vi "UDS(State).vi"() -> ()   [LabVIEW 2020]
uses:
  <vilib>/Automotive Diagnostic Command Set/Diagnostic Transport.llb/Transport Protocol Selector.ctl
  <vilib>/Automotive Diagnostic Command Set/Diagnostic Transport.llb/Property ID.ctl
  <vilib>/Automotive Diagnostic Command Set/Diagnostic Transport.llb/Diag Reference.ctl
  <vilib>/Automotive Diagnostic Command Set/Diagnostic Transport.llb/DoIP Protocol Version.ctl
  <vilib>/Automotive Diagnostic Command Set/Diagnostic Transport.llb/Diag Globals.ctl
  <vilib>/addons/Automotive Diagnostic Command Set/NI_Automotive Diagnostic Command Set.lvlib
panel:
  out "Clear DTC":bool
  out "Finish":bool
  out "Auto?":bool
  in  "Auto":bool
  in  "Reset":bool
  out "CAN_log":string[][](table)
  out "Response":u8[](array[numeric]) format="%.0x"
  in  "Close":bool
  in  "Stop":bool
  in  "Start":bool
  in  "Option":i32(ring) items=["读软件版本", "读DTC", "清DTC"]
  in  "Action":bool
  out "open_ok?":bool
  # "读软件版本→读写DTC→ 清DTC log→读软件版本→读写DTC→ 清DTC log\n运行程序，点击“Start”，Open Diagnostic\nOption：选择需要的操做；Write：手动发送指令；\nReset：清除表格内容；\nAuto：自动按照上面所要求顺序进行读写操作；\nClose：Close Diagnostic；\nStop：停止程序。"
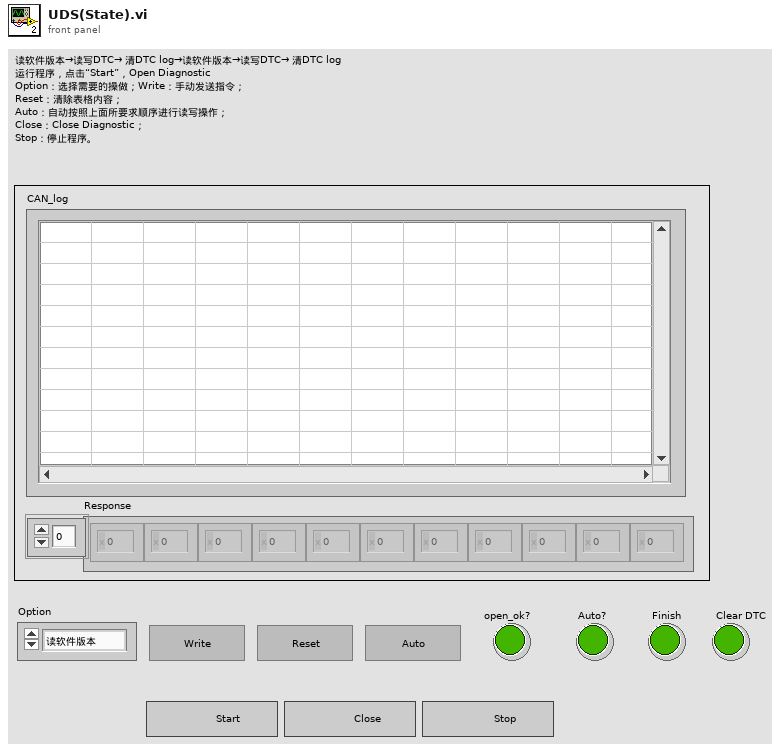
[diagram p1: front panel]
types:
  T1 = typedef "NI_Automotive Diagnostic Command Set.lvlib/Property ID.ctl" = enum16{"Timeout Diag Command", "Timeout FC (Bs)", "Timeout CF (Cr)", "Receive Block Size (BS)", "Wait Time CF (STmin)", "Max Wait Frames (N_WFTmax)", "Wait Frames to Send (N_WAIT)", "Time between Waits (T_W)", "Fill CAN Frames", "Fill Byte", "Invalid Response as Error", "Max RspPending Count", "VWTP Command Timeout", "STmin", "P2min", "Termination", "Timeout RspPending", "LIN Sleep", "Actual CAN IO Mode", "Response Plausibility Check", "Session-based Properties"}
  T2 = typedef "NI_Automotive Diagnostic Command Set.lvlib/Transport Protocol Selector.ctl" = enum16{"ISO TP - Normal Mode", "ISO TP - Mixed Mode", "VW TP 2.0", "Diagnostics on IP", "ISO TP LIN"}
  T3 = typedef "NI_Automotive Diagnostic Command Set.lvlib/Diag Reference.ctl" = cluster{"Diag CAN Handle":u32, "Transport Protocol":T2, "Receive Address Extension":u8, "Transmit Address Extension":u8, "Receive CAN Id":u32, "Transmit CAN Id":u32, "Log Frames ?":bool, "My TP Address":u8, "Other TP Address":u8, "T1":u16, "T2":u16, "T3":u16, "T4":u16, "Tx SN":u8, "Block Size":u8, "Rx SN":u8, "VW TP Initialized?":bool, "Tx block no":u8, "baud rate":u64, "Interface":string, "Channel Diag CAN Handle":u32, "UDP Connection ID":refnum<k16>, "TCP Connection ID":refnum<k5>, "Target IP Addr":u32, "Source Address":u16, "Target Address":u16, "Send Header NACK?":bool, "DLL Handle":u32, "NAD":u8, "Time Stamp read first":dbl, "Time Stamp read last":dbl, "Time Stamp write first":dbl, "Time Stamp write last":dbl, "Time Stamp write":dbl, "Time Stamp read":dbl, " I/O Mode":u32, "FD Baudrate":u64, "TX_DL":u16, "RX_DL":u16, "DoIP Protocol Version":T4, " Selected I/O Mode":u32, "TesterPresent Counter":u32, "TesterPresent Limit":u32, "TesterPresent Tick[ms]":i32, "TesterPresent RequireResponse?":bool, "TesterPresent Stored Ref?":bool, "TesterPresent Message":u8[], "TesterPresent Task Handle":i32, "TesterPresent Semaphore":T5, "Response Plausibility Check":u32, "Default Version?":bool, "Diagostic Globals":T6, "Session-based Properties?":bool}
  T4 = typedef "NI_Automotive Diagnostic Command Set.lvlib/DoIP Protocol Version.ctl" = u8
  T5 = typedef "Semaphore RefNum" = refnum<k1>
  T6 = typedef "NI_Automotive Diagnostic Command Set.lvlib/Diag Globals.ctl" = cluster{"Timeout FC (Bs)":u32, "Timeout CF (Cr)":u32, "Timeout Diag Command":u32, "Receive Block Size (BS)":u8, "Wait Time CF (STmin)":u8, "Max Waits (N_WFTmax)":u8, "Waits to Send (N_WAIT)":i32, "Time between Waits (TW)":u32, "Fill CAN Frames?":bool, "Fill Byte":u32, "Invalid Response as Error?":bool, "Max RspPending Count":u32, "VWTP Command Timeout":u32, "Transport Protocol":T2, "Diag CAN Handle":u32, "DLL Handle":u32, "Timeout RspPending":u32}
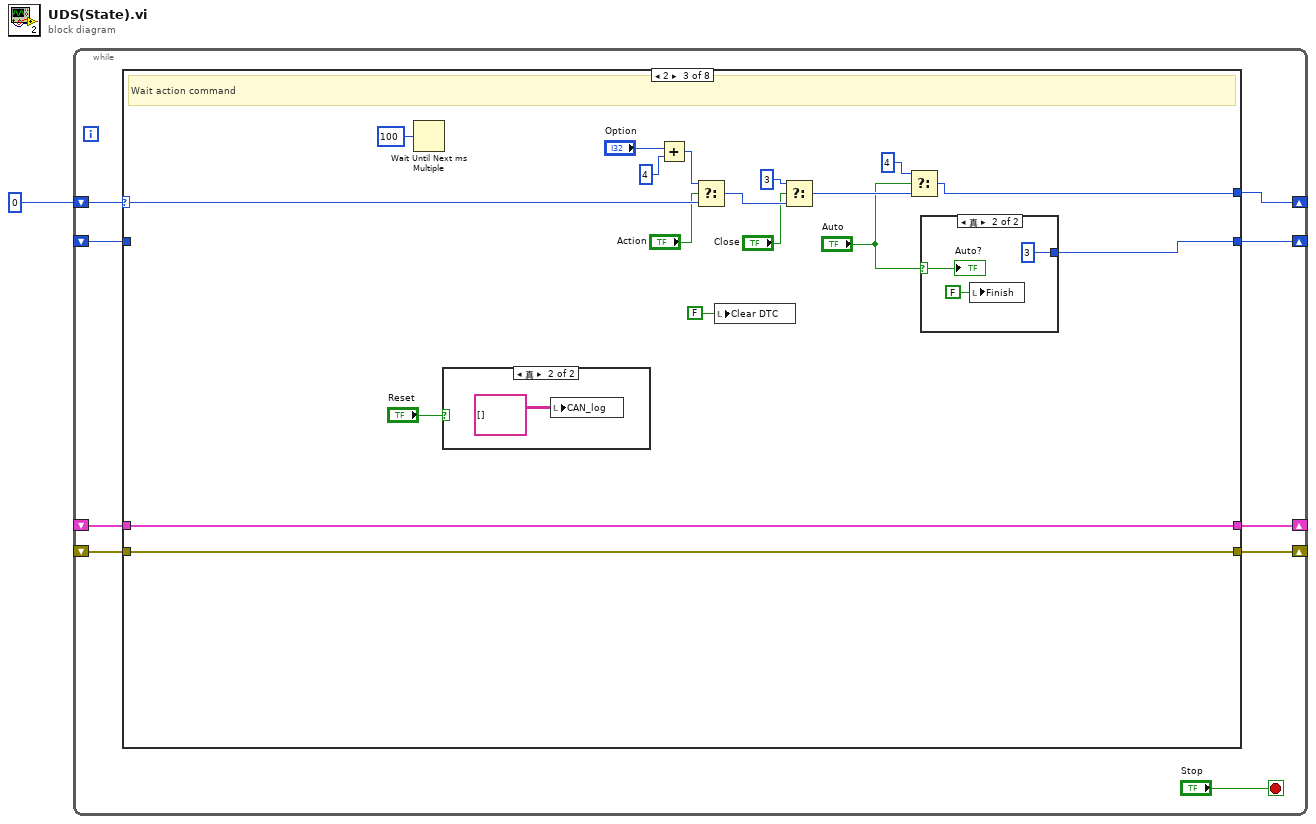
[diagram p0: block diagram]
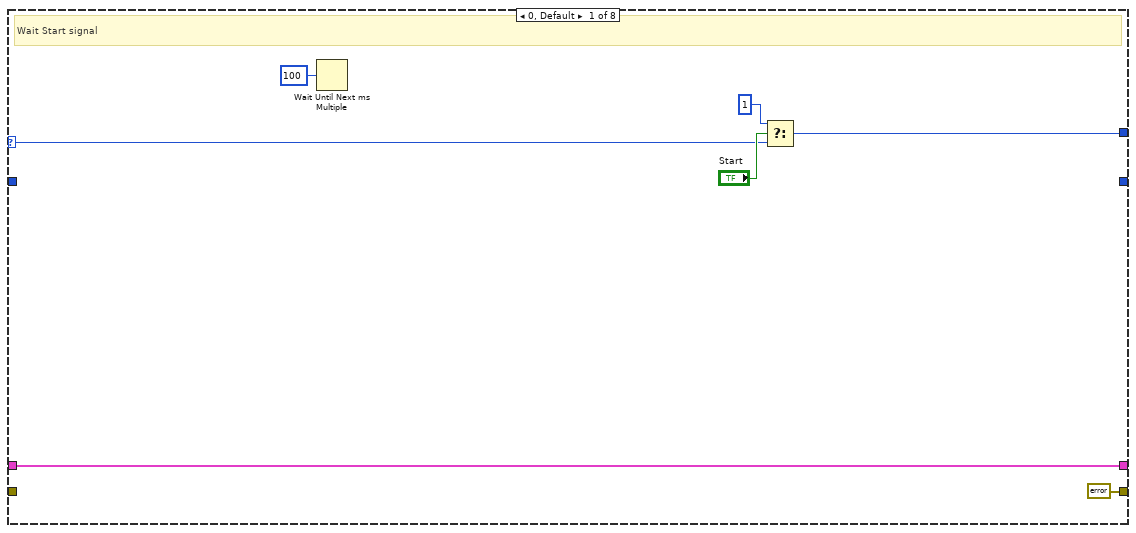
[diagram p2: hidden frame]
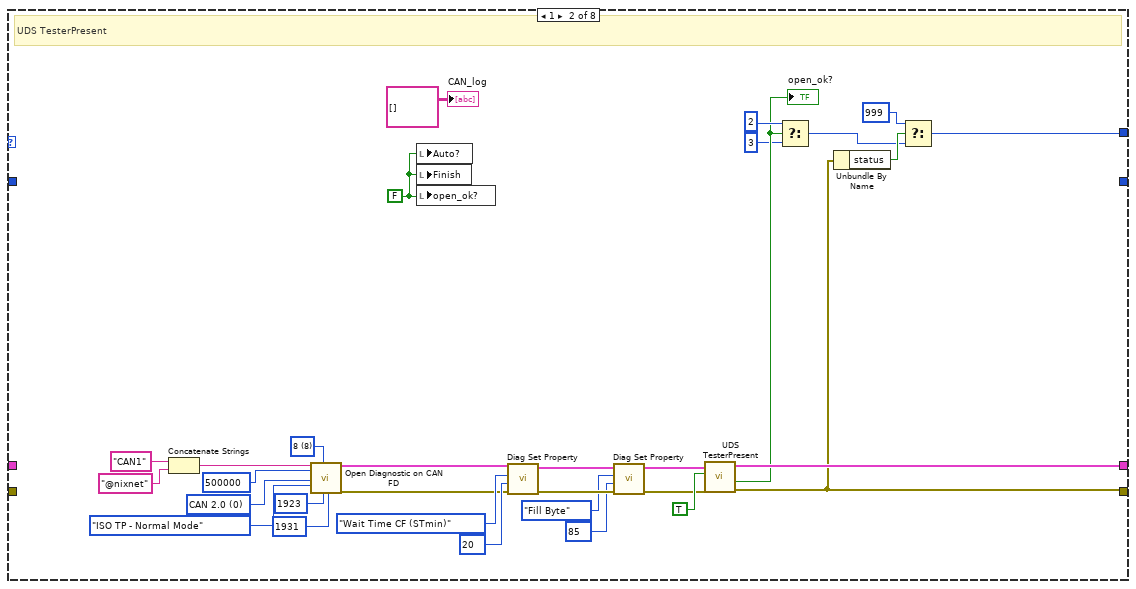
[diagram p3: hidden frame]
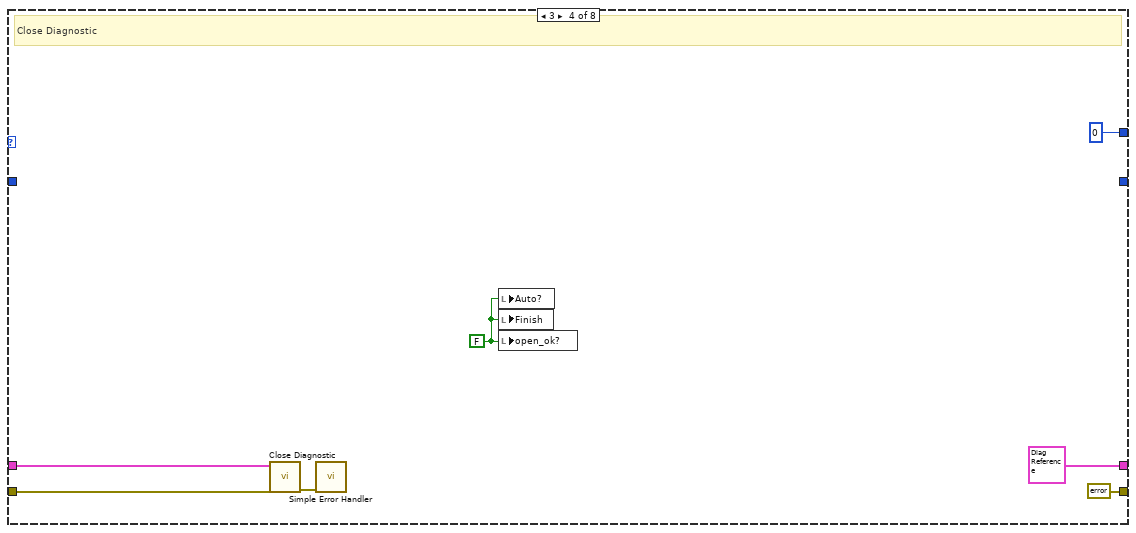
[diagram p6: hidden frame]
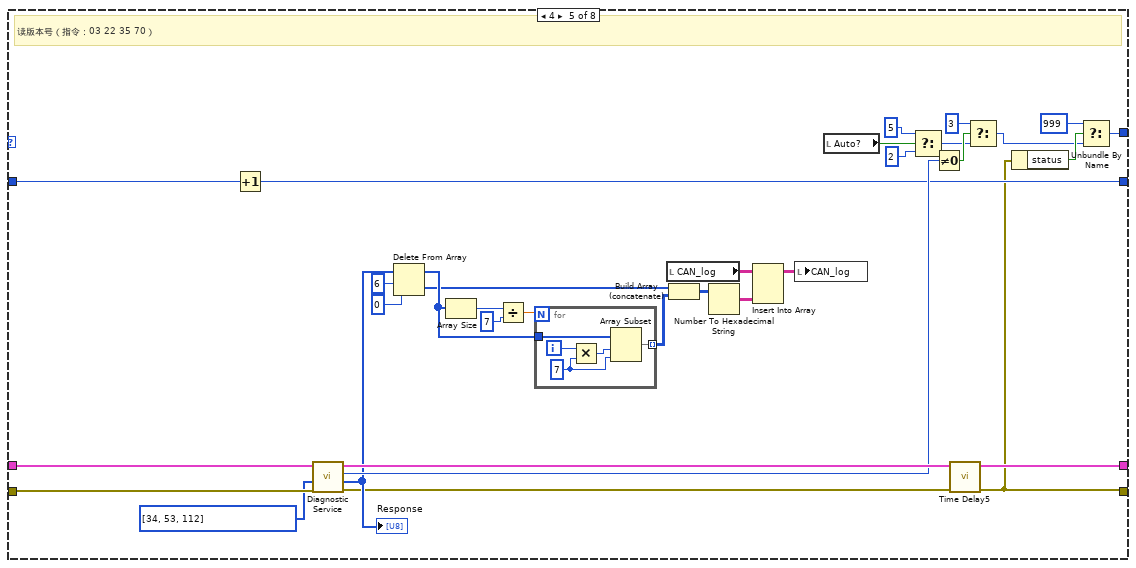
[diagram p7: hidden frame]
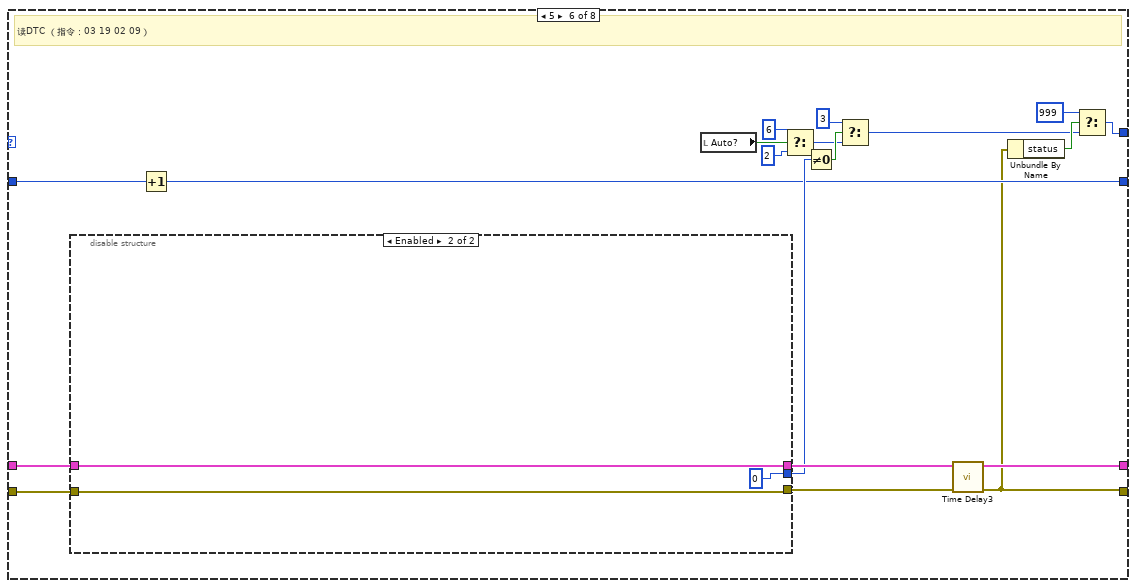
[diagram p8: hidden frame]
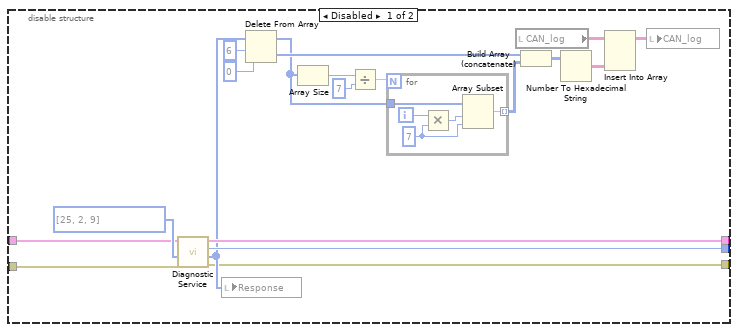
[diagram p9: hidden frame]
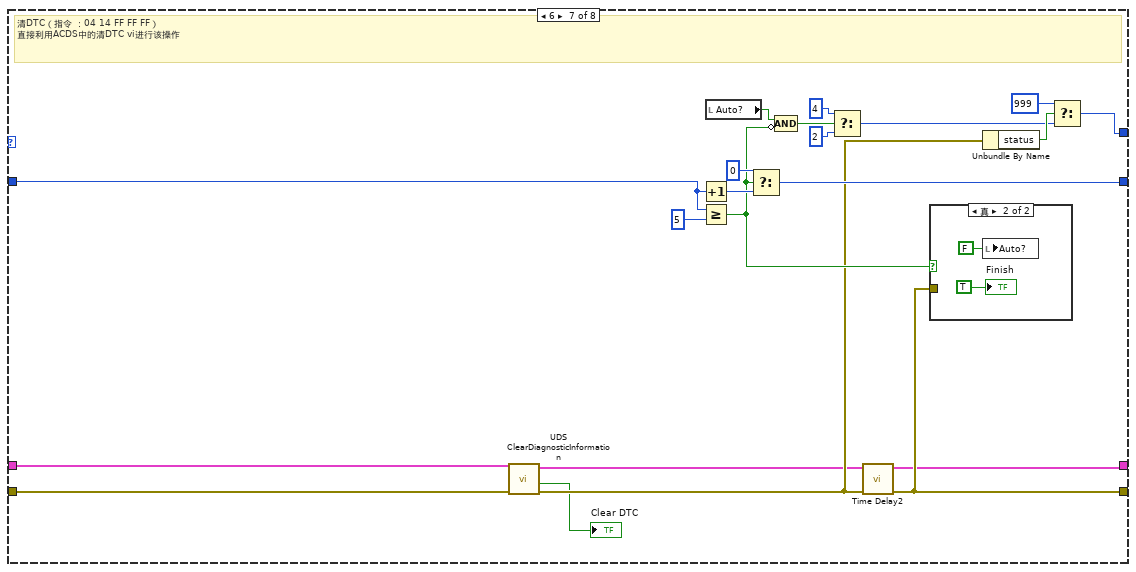
[diagram p10: hidden frame]
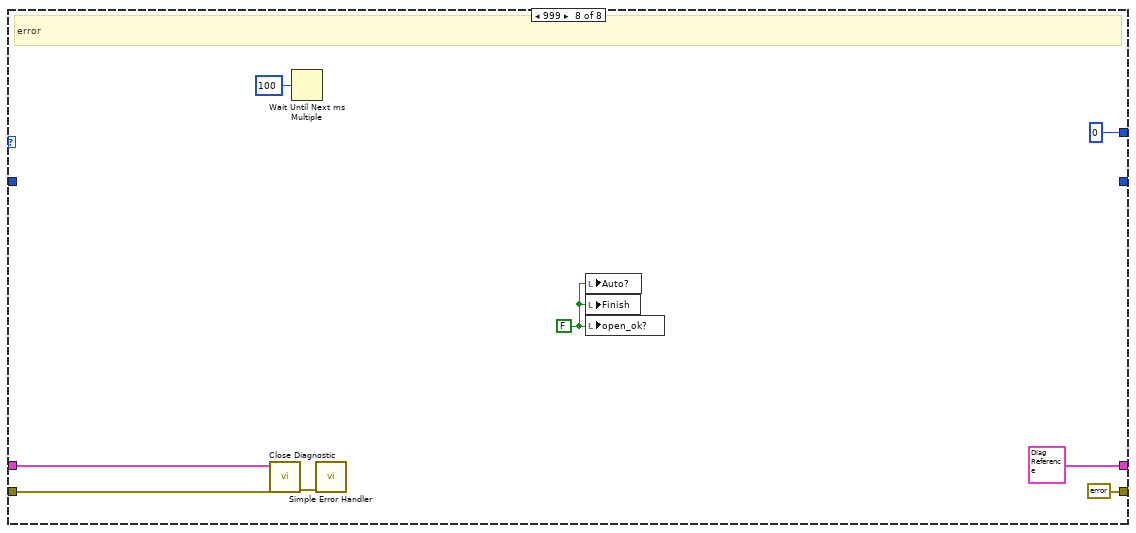
[diagram p12: hidden frame]
diagram:
  n1 = while {
    shift-right: [w5] -> _
    shift-left: 0 -> [w10]
    shift-right: [w7] -> _
    shift-left: _ -> [w9]
    shift-right: [w6] -> _
    shift-left: _ -> [w8]
    shift-right: [w3] -> _
    shift-left: _ -> [w2]
    stop <- "Stop" stop-if-true
    n2 = case shown="2" w10 {
      selector: w10 -> [w13 _ w66 _ _ _ _ _]
      tunnel: w9 -> [w17 _ w65 w75 w109 w131 w164 w187]
      tunnel: w8 -> [_ _ w64 w76 w81 w130 w163 w188]
      tunnel: [w17 w48 w65 T3 {"Diag CAN Handle"=0, "Transport Protocol"=enum."ISO TP - Normal Mode", "Receive Address Extension"=0, "Transmit Address Extension"=0, "Receive CAN Id"=0, "Transmit CAN Id"=0, "Log Frames ?"=FALSE, "My TP Address"=0, "Other TP Address"=0, "T1"=0, "T2"=0, "T3"=0, "T4"=0, "Tx SN"=0, "Block Size"=0, "Rx SN"=0, "VW TP Initialized?"=FALSE, "Tx block no"=0, "baud rate"=0, "Interface"="", "Channel Diag CAN Handle"=0, "UDP Connection ID"=refnum, "TCP Connection ID"=refnum, "Target IP Addr"=0, "Source Address"=0, "Target Address"=0, "Send Header NACK?"=FALSE, "DLL Handle"=0, "NAD"=0, "Time Stamp read first"=0.0, "Time Stamp read last"=0.0, "Time Stamp write first"=0.0, "Time Stamp write last"=0.0, "Time Stamp write"=0.0, "Time Stamp read"=0.0, " I/O Mode"=0, "FD Baudrate"=0, "TX_DL"=8, "RX_DL"=8, "DoIP Protocol Version"=1, " Selected I/O Mode"=0, "TesterPresent Counter"=0, "TesterPresent Limit"=0, "TesterPresent Tick[ms]"=10, "TesterPresent RequireResponse?"=FALSE, "TesterPresent Stored Ref?"=FALSE, "TesterPresent Message"=[], "TesterPresent Task Handle"=0, "TesterPresent Semaphore"=refnum, "Response Plausibility Check"=1, "Default Version?"=TRUE, "Diagostic Globals"={"Timeout FC (Bs)"=250, "Timeout CF (Cr)"=250, "Timeout Diag Command"=1000, "Receive Block Size (BS)"=0, "Wait Time CF (STmin)"=5, "Max Waits (N_WFTmax)"=10, "Waits to Send (N_WAIT)"=0, "Time between Waits (TW)"=25, "Fill CAN Frames?"=TRUE, "Fill Byte"=255, "Invalid Response as Error?"=FALSE, "Max RspPending Count"=5, "VWTP Command Timeout"=50, "Transport Protocol"=enum."Diagnostics on IP", "Diag CAN Handle"=0, "DLL Handle"=0, "Timeout RspPending"=1000}, "Session-based Properties?"=FALSE} ("diag ref out") w108 w129 w161 T3 {"Diag CAN Handle"=0, "Transport Protocol"=enum."ISO TP - Normal Mode", "Receive Address Extension"=0, "Transmit Address Extension"=0, "Receive CAN Id"=0, "Transmit CAN Id"=0, "Log Frames ?"=FALSE, "My TP Address"=0, "Other TP Address"=0, "T1"=0, "T2"=0, "T3"=0, "T4"=0, "Tx SN"=0, "Block Size"=0, "Rx SN"=0, "VW TP Initialized?"=FALSE, "Tx block no"=0, "baud rate"=0, "Interface"="", "Channel Diag CAN Handle"=0, "UDP Connection ID"=refnum, "TCP Connection ID"=refnum, "Target IP Addr"=0, "Source Address"=0, "Target Address"=0, "Send Header NACK?"=FALSE, "DLL Handle"=0, "NAD"=0, "Time Stamp read first"=0.0, "Time Stamp read last"=0.0, "Time Stamp write first"=0.0, "Time Stamp write last"=0.0, "Time Stamp write"=0.0, "Time Stamp read"=0.0, " I/O Mode"=0, "FD Baudrate"=0, "TX_DL"=8, "RX_DL"=8, "DoIP Protocol Version"=1, " Selected I/O Mode"=0, "TesterPresent Counter"=0, "TesterPresent Limit"=0, "TesterPresent Tick[ms]"=10, "TesterPresent RequireResponse?"=FALSE, "TesterPresent Stored Ref?"=FALSE, "TesterPresent Message"=[], "TesterPresent Task Handle"=0, "TesterPresent Semaphore"=refnum, "Response Plausibility Check"=1, "Default Version?"=TRUE, "Diagostic Globals"={"Timeout FC (Bs)"=250, "Timeout CF (Cr)"=250, "Timeout Diag Command"=1000, "Receive Block Size (BS)"=0, "Wait Time CF (STmin)"=5, "Max Waits (N_WFTmax)"=10, "Waits to Send (N_WAIT)"=0, "Time between Waits (TW)"=25, "Fill CAN Frames?"=TRUE, "Fill Byte"=255, "Invalid Response as Error?"=FALSE, "Max RspPending Count"=5, "VWTP Command Timeout"=50, "Transport Protocol"=enum."Diagnostics on IP", "Diag CAN Handle"=0, "DLL Handle"=0, "Timeout RspPending"=1000}, "Session-based Properties?"=FALSE} ("diag ref out")] -> w7
      tunnel: [errorcluster {"status"=FALSE, "code"=0, "source"=""} ("error out") w35 w64 errorcluster {"status"=FALSE, "code"=0, "source"=""} ("error out") w79 w115 w165 errorcluster {"status"=FALSE, "code"=0, "source"=""} ("error out")] -> w6
      tunnel: [w12 w31 w51 0 ("t") w95 w117 w166 0 ("t")] -> w5
      tunnel: [_ _ w52 _ w101 w122 w177 _] -> w3
      tunnel: w2 -> [_ _ _ _ w100 w123 w176 _]
      frame 0, Default {
        # "Wait Start signal"
        n3 = Wait Until Next ms Multiple(millisecond multiple=u32 100) -> ()  [unwired: 1 out]
        n4 = Select(t=1, s="Start", f=w13) -> (s? t:f=w12:i32)
      }
      frame 1 {
        w29 = FALSE ("success?")
        w41 = u16 8 items=["8"=8, "12"=12, "16"=16, "20"=20, "24"=24, "32"=32, "48"=48, "64"=64] ("Max DLC")
        w43 = u32 0 items=["CAN 2.0", "CAN FD", "CAN FD+BRS", "ECU Determined"] ("IO Mode")
        # "UDS TesterPresent"
        n5 = Concatenate Strings("CAN1" ("Name"), "@nixnet") -> (w45:string)
        n6 = call <vilib>:"Open Diagnostic on CAN FD.vi"("CAN Interface"=w45, "Baud Rate"=u64 500000, "IO Mode"=w43, "Transport Protocol"=Transport_Protocol_Selector."ISO TP - Normal Mode", "Max DLC"=w41, "Transmit ID"=u32 1923, "Receive ID"=u32 1931) -> ("diag ref out"=w21:T3, "error out"=w19:errorcluster)  [unwired: 11 in]
        n7 = local write "Auto?"(w29) -> ()
        n8 = local write "Finish"(w29) -> ()
        n9 = local write "open_ok?"(w29) -> ()
        n10 = call <vilib>:"Diag Set Property.vi"("error in (no error)"=w19, "property value"=u32 20, "property ID"=Property_ID."Wait Time CF (STmin)", "diag ref in"=w21) -> ("error out"=w27:errorcluster, "diag ref out"=w26:T3)  [unwired: 6 in]
        n11 = call <vilib>:"Diag Set Property.vi"("error in (no error)"=w27, "property value"=u32 85, "property ID"=Property_ID."Fill Byte", "diag ref in"=w26) -> ("error out"=w18:errorcluster, "diag ref out"=w20:T3)  [unwired: 6 in]
        n12 = call <vilib>:"UDS TesterPresent.vi"("error in (no error)"=w18, "response required?"=TRUE, "diag ref in"=w20) -> ("error out"=w35:errorcluster, "success?"=w46:bool, "diag ref out"=w48:T3)  [unwired: 6 out]
        "open_ok?" <- w46
        n13 = Select(t=2, s=w46, f=3) -> (s? t:f=w32:i32)
        n14 = Unbundle By Name(w35) -> ("status"=w34:bool)
        n15 = Select(t=999, s=w34, f=w32) -> (s? t:f=w31:i32)
        "CAN_log" <- string[][] [] ("Table")
      }
      frame 2 {
        # "Wait action command"
        n16 = Wait Until Next ms Multiple(millisecond multiple=u32 100) -> ()  [unwired: 1 out]
        n17 = case shown="真" "Reset" {
          frame False {
          }
          frame True {
            n18 = local write "CAN_log"(string[][] [] ("Table")) -> ()
          }
        }
        n19 = Add(x="Option", y=4) -> (x+y=w57:i32)
        n20 = Select(t=w57, s="Action", f=w66) -> (s? t:f=w62:i32)
        n21 = local write "Clear DTC"(FALSE ("Clear DTC")) -> ()
        n22 = Select(t=3, s="Close", f=w62) -> (s? t:f=w55:i32)
        n23 = Select(t=4, s="Auto", f=w55) -> (s? t:f=w51:i32)
        n24 = case shown="真" "Auto" {
          selector: "Auto" -> [_ w69]
          tunnel: [_ 3] -> w52
          frame False {
          }
          frame True {
            n25 = local write "Finish"(FALSE ("Finish")) -> ()
            "Auto?" <- w69
          }
        }
      }
      frame 3 {
        w71 = FALSE ("success?")
        # "Close Diagnostic"
        n26 = call <vilib>:"Close Diagnostic.vi"("error in (no error)"=w76, "diag ref in"=w75) -> ("error out"=w77:errorcluster)  [unwired: 9 out]
        n27 = call <vilib>:"Simple Error Handler.vi"("error in (no error)"=w77) -> ()  [unwired: 1 in, 8 out]
        n28 = local write "Auto?"(w71) -> ()
        n29 = local write "Finish"(w71) -> ()
        n30 = local write "open_ok?"(w71) -> ()
      }
      frame 4 {
        # "读版本号（指令：03 22 35 70）"
        n31 = Increment(x=w100) -> (x+1=w101:i32)
        n32 = call <vilib>:"Diagnostic Service.vi"("error in (no error)"=w81, "data in"=u8[] [34, 53, 112] ("Request"), "diag ref in"=w109) -> ("error out"=w80:errorcluster, "data out"=w94:u8[], "error code"=w107:u8, "diag ref out"=w108:T3)  [unwired: 1 in, 4 out]
        "Response" <- w94
        n33 = Delete From Array(array=w94, length=6, index=0) -> (deleted portion=w82:u8[], array with subset deleted=w88:u8[])
        n34 = Array Size(array=w88) -> (size(s)=w91:i32)
        n35 = Divide(x=w91, y=7) -> (x/y=w89:dbl)
        n36 = for {
          N: w89 -> [_]
          tunnel: w88 -> [w114]
          tunnel: [w110] -> w87 mode=indexing
          i -> [w112]
          w113 = 7 ("length")
          n37 = Multiply(x=w112, y=w113) -> (x*y=w111:i32)
          n38 = Array Subset(array=w114, index=w111, length=w113) -> (w110:u8[])
        }
        n39 = local read "CAN_log"() -> (w86:string[][])
        n40 = Build Array (concatenate)(w82, w87) -> (w84:u8[][])
        n41 = Number To Hexadecimal String(2:w84) -> (0:w83:string[][])  [unwired: 1 in]
        n42 = Insert Into Array(array=w86, new element=w83) -> (w85:string[][])  [unwired: 2 in]
        n43 = local write "CAN_log"(w85) -> ()
        n44 = local read "Auto?"() -> (w104:bool)
        n45 = Select(t=5, s=w104, f=2) -> (s? t:f=w103:i32)
        n46 = Not Equal To 0?(x=w107) -> (x != 0?=w105:bool)
        n47 = call "Time Delay5"("error in (no error)"=w80) -> ("error out"=w79:errorcluster)  [unwired: 10 in]
        n48 = Select(t=3, s=w105, f=w103) -> (s? t:f=w96:i32)
        n49 = Unbundle By Name(w79) -> ("status"=w98:bool)
        n50 = Select(t=999, s=w98, f=w96) -> (s? t:f=w95:i32)
      }
      frame 5 {
        # "读DTC （指令：03 19 02 09）"
        n51 = disable-structure shown="Enabled" {
          disable-tunnel: w131 -> [w150 w158]
          disable-tunnel: w130 -> [w149 w157]
          disable-tunnel: [w148 w158] -> w129
          disable-tunnel: [w147 u8 0 ("error code")] -> w127
          disable-tunnel: [w133 w157] -> w116
          frame Disabled {
            n52 = call <vilib>:"Diagnostic Service.vi"("error in (no error)"=w149, "data in"=u8[] [25, 2, 9] ("Request"), "diag ref in"=w150) -> ("error out"=w133:errorcluster, "data out"=w137:u8[], "error code"=w147:u8, "diag ref out"=w148:T3)  [unwired: 1 in, 4 out]
            n53 = local write "Response"(w137) -> ()
            n54 = Delete From Array(array=w137, length=6, index=0) -> (deleted portion=w141:u8[], array with subset deleted=w134:u8[])
            n55 = Array Size(array=w134) -> (size(s)=w146:i32)
            n56 = Divide(x=w146, y=7) -> (x/y=w145:dbl)
            n57 = for {
              N: w145 -> [_]
              tunnel: w134 -> [w152]
              tunnel: [w153] -> w136 mode=indexing
              i -> [w155]
              w156 = 7 ("length")
              n58 = Multiply(x=w155, y=w156) -> (x*y=w154:i32)
              n59 = Array Subset(array=w152, index=w154, length=w156) -> (w153:u8[])
            }
            n60 = local read "CAN_log"() -> (w144:string[][])
            n61 = Build Array (concatenate)(w141, w136) -> (w135:u8[][])
            n62 = Number To Hexadecimal String(2:w135) -> (0:w142:string[][])  [unwired: 1 in]
            n63 = Insert Into Array(array=w144, new element=w142) -> (w143:string[][])  [unwired: 2 in]
            n64 = local write "CAN_log"(w143) -> ()
          }
          frame Enabled {
          }
        }
        n65 = Increment(x=w123) -> (x+1=w122:i32)
        n66 = local read "Auto?"() -> (w126:bool)
        n67 = Select(t=6, s=w126, f=2) -> (s? t:f=w124:i32)
        n68 = Not Equal To 0?(x=w127) -> (x != 0?=w128:bool)
        n69 = Select(t=3, s=w128, f=w124) -> (s? t:f=w118:i32)
        n70 = call "Time Delay3"("error in (no error)"=w116) -> ("error out"=w115:errorcluster)  [unwired: 10 in]
        n71 = Unbundle By Name(w115) -> ("status"=w120:bool)
        n72 = Select(t=999, s=w120, f=w118) -> (s? t:f=w117:i32)
      }
      frame 6 {
        # "清DTC（指令 ：04 14 FF FF FF）\n直接利用ACDS中的清DTC vi进行该操作"
        n73 = call <vilib>:"UDS ClearDiagnosticInformation.vi"("error in (no error)"=w163, "diag ref in"=w164) -> ("error out"=w162:errorcluster, "success?"=→"Clear DTC":bool, "diag ref out"=w161:T3)  [unwired: 7 in]
        n74 = Increment(x=w176) -> (x+1=w175:i32)
        n75 = Greater Or Equal?(x=w176, y=5) -> (x >= y?=w170:bool)
        n76 = local read "Auto?"() -> (w173:bool)
        n77 = Select(t=0, s=w170, f=w175) -> (s? t:f=w177:i32)
        n78 = Compound Arithmetic op=AND(w173, invert w170) -> (w172:bool)
        n79 = Select(t=4, s=w172, f=2) -> (s? t:f=w167:i32)
        n80 = call "Time Delay2"("error in (no error)"=w162) -> ("error out"=w165:errorcluster)  [unwired: 10 in]
        n81 = case shown="真" w170 {
          tunnel: w165 -> [_ _]
          frame False {
          }
          frame True {
            n82 = local write "Auto?"(FALSE ("Auto?")) -> ()
            "Finish" <- TRUE ("Finish")
          }
        }
        n83 = Unbundle By Name(w162) -> ("status"=w169:bool)
        n84 = Select(t=999, s=w169, f=w167) -> (s? t:f=w166:i32)
      }
      frame 999 {
        w183 = FALSE ("success?")
        # "error"
        n85 = call <vilib>:"Close Diagnostic.vi"("error in (no error)"=w188, "diag ref in"=w187) -> ("error out"=w189:errorcluster)  [unwired: 9 out]
        n86 = Wait Until Next ms Multiple(millisecond multiple=u32 100) -> ()  [unwired: 1 out]
        n87 = call <vilib>:"Simple Error Handler.vi"("error in (no error)"=w189) -> ()  [unwired: 1 in, 8 out]
        n88 = local write "Auto?"(w183) -> ()
        n89 = local write "Finish"(w183) -> ()
        n90 = local write "open_ok?"(w183) -> ()
      }
    }
  }
